vi "LKIF_ClearFigureData.vi"(8 "error in (no error)":errorcluster {"code" format="%x"}) -> (0 "error out":errorcluster {"code" format="%x"})   [LabVIEW 8.6, in "Keyence LK-G3000.lvlib"]
uses:
  Keyence LK-G3000.lvlib
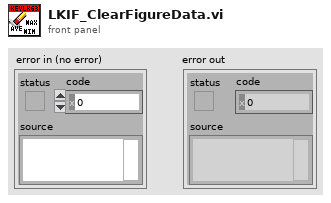
[diagram p1: front panel]
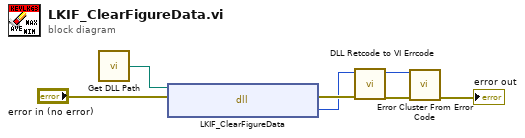
[diagram p0: block diagram]
diagram:
  n1 = call "Get DLL Path.vi"() -> ("DLL Path"=w3:path)  [unwired: 1 in]
  n2 = dll-call lib="C:/Program Files/National Instruments/LabVIEW 2011/instr.lib/Keyence LK-G3000/LkIF.dll" fn="LKIF_ClearFigureData"(path in=w3, error in="error in (no error)") -> (error out=w5:errorcluster, "RC"=w4:i32)  [unwired: 1 in, 1 out]
  n3 = call "DLL Retcode to VI Errcode.vi"("error in (no error)"=w5, "DLL Retcode"=w4) -> ("error out"=w7:errorcluster, "VI Errcode"=w6:i32)  [unwired: 8 in]
  n4 = call <vilib>:"Error Cluster From Error Code.vi"("error in (no error)"=w7, "error code (0)"=w6) -> ("error out"=→"error out":errorcluster)  [unwired: 7 in]
